vi "Decode 4134 Event.vi"(0 "4134 Event":u8) -> (1 "Event Type":T3(ring), 2 "NXT Button":T1(ring), 3 "FTC Button":T2(ring), 4 "Source":enum16{"NXT", "Remote 1", "Remote 2"}(ring))   [LabVIEW 2012, in "FTC.lvlib" / "Remote Interface.lvlib"]
uses:
  Remote Interface.lvlib
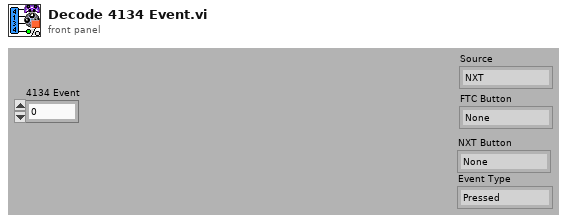
[diagram p1: front panel]
types:
  T1 = enum16{"None", "Left Button", "Right Button", "Enter Button"}
  T2 = enum16{"None", "Button 1", "Button 2", "Button 3", "Button 4", "Button 5", "Button 6", "Button 7", "Button 8", "Button 9", "Button 10", "Button 11", "Button 12", "POV Up", "POV Up Right", "POV Right", "POV Down Right", "POV Down", "POV Down Left", "POV Left", "POV Up Left"}
  T3 = enum16{"Pressed", "Released", "Toggled", "Untoggled"}
  T4 = enum16{"1-1", "1-2", "1-3", "1-4", "1-5", "1-6", "1-7", "1-8", "1-9", "1-10", "1-11", "1-12", "2-1", "2-2", "2-3", "2-4", "2-5", "2-6", "2-7", "2-8", "2-9", "2-10", "2-11", "2-12", "NXT-L", "NXT-R", "NXT-E", "1-U", "1-UR", "1-R", "1-DR", "1-D", "1-DL", "1-L", "1-UL", "2-U", "2-UR", "2-R", "2-DR", "2-D", "2-DL", "2-L", "2-UL"}
  T5 = enum8{"Pressed", "Released", "Toggled", "Untoggled"}
  T6 = enum8{"1-1", "1-2", "1-3", "1-4", "1-5", "1-6", "1-7", "1-8", "1-9", "1-10", "1-11", "1-12", "2-1", "2-2", "2-3", "2-4", "2-5", "2-6", "2-7", "2-8", "2-9", "2-10", "2-11", "2-12", "NXT-L", "NXT-R", "NXT-E", "1-U", "1-UR", "1-R", "1-DR", "1-D", "1-DL", "1-L", "1-UL", "2-U", "2-UR", "2-R", "2-DR", "2-D", "2-DL", "2-L", "2-UL"}
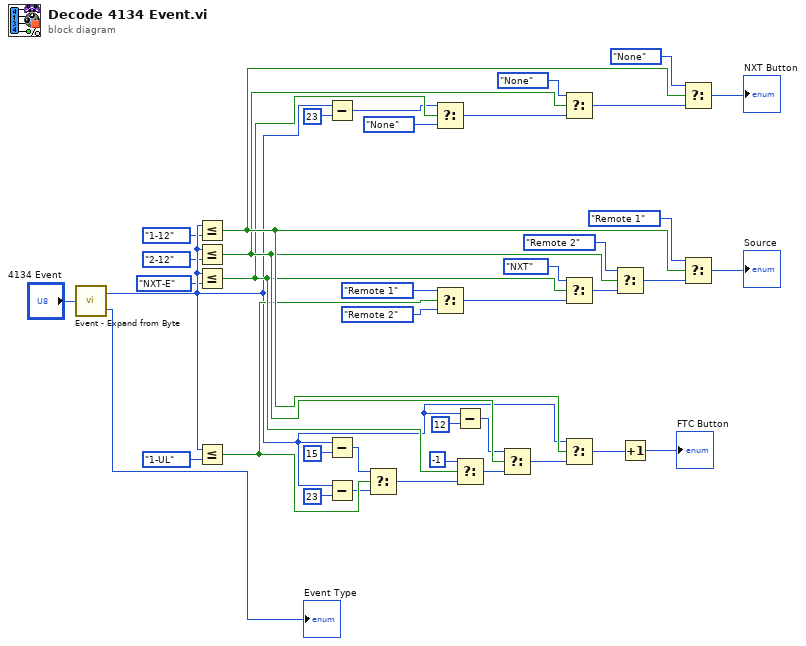
[diagram p0: block diagram]
diagram:
  n1 = call "Event - Expand from Byte.vi"("8-bit event"="4134 Event") -> ("4134 Event Type"=→"Event Type":T5, "4134 Button ID"=w34:T6)
  n2 = Less Or Equal?(x=w34, y=T4."1-12") -> (x <= y?=w39:bool)
  n3 = Less Or Equal?(x=w34, y=T4."2-12") -> (x <= y?=w38:bool)
  n4 = Less Or Equal?(x=w34, y=T4."NXT-E") -> (x <= y?=w37:bool)
  n5 = Less Or Equal?(x=w34, y=T4."1-UL") -> (x <= y?=w36:bool)
  n6 = Subtract(x=w34, y=23) -> (x-y=w7:i32)
  n7 = Subtract(x=w34, y=15) -> (x-y=w26:i32)
  n8 = Subtract(x=w34, y=23) -> (x-y=w24:i32)
  n9 = Select(t=w26, s=w36, f=w24) -> (s? t:f=w28:i32)
  n10 = Select(t=w7, s=w37, f=T1."None" ("NXT Button")) -> (s? t:f=w6:i32)
  n11 = Select(t=enum16{"NXT", "Remote 1", "Remote 2"}."Remote 1" ("Source"), s=w36, f=enum16{"NXT", "Remote 1", "Remote 2"}."Remote 2" ("Source")) -> (s? t:f=w15:enum16{"NXT", "Remote 1", "Remote 2"})
  n12 = Subtract(x=w34, y=12) -> (x-y=w22:i32)
  n13 = Select(t=-1, s=w37, f=w28) -> (s? t:f=w30:i32)
  n14 = Select(t=w22, s=w38, f=w30) -> (s? t:f=w33:i32)
  n15 = Select(t=T1."None" ("NXT Button"), s=w38, f=w6) -> (s? t:f=w10:i32)
  n16 = Select(t=enum16{"NXT", "Remote 1", "Remote 2"}."NXT" ("Source"), s=w37, f=w15) -> (s? t:f=w20:enum16{"NXT", "Remote 1", "Remote 2"})
  n17 = Select(t=w34, s=w39, f=w33) -> (s? t:f=w32:i32)
  n18 = Select(t=enum16{"NXT", "Remote 1", "Remote 2"}."Remote 2" ("Source"), s=w38, f=w20) -> (s? t:f=w21:enum16{"NXT", "Remote 1", "Remote 2"})
  n19 = Increment(x=w32) -> (x+1=→"FTC Button":i32)
  n20 = Select(t=T1."None" ("NXT Button"), s=w39, f=w10) -> (s? t:f=→"NXT Button":i32)
  n21 = Select(t=enum16{"NXT", "Remote 1", "Remote 2"}."Remote 1" ("Source"), s=w39, f=w21) -> (s? t:f=→"Source":enum16{"NXT", "Remote 1", "Remote 2"})
